vi "S2C_FORNAX_Proc_FindFnxMsg.vi"(8 "Error In":errorcluster, 11 "MsgName":string) -> (0 "Error Out":errorcluster, 3 "Message":string)   [LabVIEW 2015]
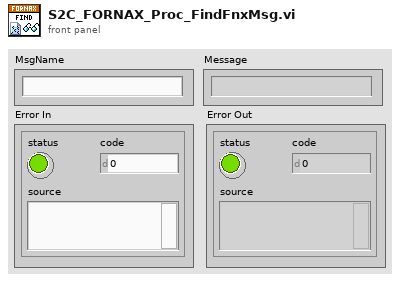
[diagram p1: front panel]
types:
  T1 = cluster{"RawMsg":string, "ViperMsg":string[], "DDSMsg":string[]}
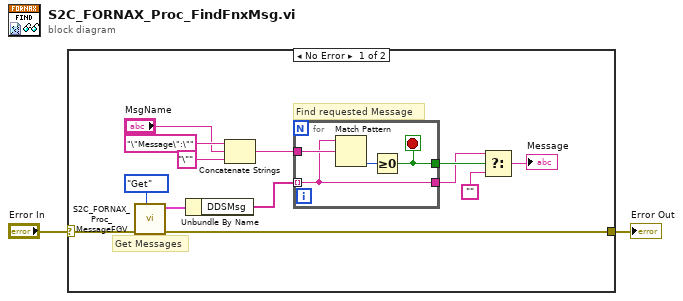
[diagram p0: block diagram]
diagram:
  n1 = case shown="No Error" "Error In" {
    selector: "Error In" -> [w15 w20]
    tunnel: [w7 w20] -> w1
    frame No Error {
      # "Find requested Message"
      # "Get Messages"
      n2 = call "S2C_FORNAX_Proc_MessageFGV.vi"("Action"=enum16{"Set", "Get"}."Get", "Error In"=w15) -> ("Error Out"=w7:errorcluster, "Msg Out"=w10:T1)  [unwired: 8 in]
      n3 = Unbundle By Name(w10) -> ("DDSMsg"=w9:string[])
      n4 = Concatenate Strings("\"Message\":\"" ("regular expression"), "MsgName", "\"" ("regular expression")) -> (w8:string)
      n5 = for {
        tunnel: w9 -> [w17] mode=indexing
        tunnel: w8 -> [w19]
        tunnel: [w17] -> w5
        tunnel: [w16] -> w6
        stop <- w16 stop-if-true
        n6 = Match Pattern(string=w17, regular expression=w19) -> (offset past match=w18:i32)  [unwired: 1 in, 3 out]
        n7 = Greater Or Equal To 0?(x=w18) -> (x >= 0?=w16:bool)
      }
      n8 = Select(t=w5, s=w6, f="") -> (s? t:f=→"Message":string)
    }
    frame Error {
    }
  }
  "Error Out" <- w1
